vi "HFRR ADV v04.vi"() -> ()   [LabVIEW 2025] (continued)
              n1887 = local write "Com Port 1"(w2844) -> ()
            }
            frame 5 {
              n1888 = local write "visa due"(w2845) -> ()
              n1889 = local write "Com Port 2"(w2845) -> ()
            }
            frame 6 {
              n1890 = String To Path(string=w2846) -> (path=w2847:path)
              n1891 = local write "File Path"(w2847) -> ()
              "String" <- w2846
            }
            frame 7 {
              n1892 = local write "DISPLACEMENT :"(w2848) -> ()
            }
            frame 8 {
              n1893 = local write "STROKE GAIN :"(w2849) -> ()
            }
            frame 9 {
              n1894 = local read "Stroke PID Gains"() -> (w2852:T8)
              n1895 = Bundle By Name(cluster=w2852, "Proportional Gain (Kc)"=w2850) -> (w2851:T8)
              n1896 = local write "Stroke PID Gains"(w2851) -> ()
            }
            frame 10 {
              n1897 = local write "Language Selection"(w2853) -> ()
            }
            frame 11 {
              n1898 = local write "CH-POWER +"(w2854) -> ()
            }
            frame 12 {
              n1899 = local write "CH-POWER -"(w2855) -> ()
            }
            frame 13 {
              n1900 = local write "CH-HEATER"(w2856) -> ()
            }
            frame 14 {
              n1901 = local write "CH-HUMIDITY WET"(w2857) -> ()
            }
            frame 15 {
              n1902 = local write "CH-HUMIDITY DRY"(w2858) -> ()
            }
            frame 16 {
              n1903 = local read "Stroke PID Gains"() -> (w2861:T8)
              n1904 = Bundle By Name(cluster=w2861, "Integral Time (Ti, min)"=w2859) -> (w2860:T8)
              n1905 = local write "Stroke PID Gains"(w2860) -> ()
            }
            frame 17 {
              n1906 = local write "AIR TEMP INTERCEPT:"(w2862) -> ()
            }
            frame 18 {
              n1907 = local write "TEMP INTERCEPT:"(w2863) -> ()
            }
            frame 19 {
              n1908 = local write "S.NO"(w2864) -> ()
            }
            frame 20 {
              n1909 = local write "Com Port 3"(w2865) -> ()
            }
            frame 21 {
              n1910 = local write "LvdtOff"(w2866) -> ()
            }
            frame 22, Default {
            }
          }
        }
      }
    }
    n1911 = case shown="True" w2808 {
      frame False {
        # "79.77669138"
        # "2.3554"
        n1912 = local read "FRIC. FORCE :"() -> (w2871:dbl)
        n1913 = local read "FF cal val"() -> (w2868:dbl[])
        n1914 = Multiply(x=w2871, y=79.77669138) -> (x*y=w2870:dbl)
        n1915 = Multiply(x=w2868, y=w2870) -> (x*y=→"FF Calibration g":dbl[])
        "Err Count" <- 0 ("y")
      }
      frame True {
        n1916 = stacked-sequence {
          frame #0 {
            n1917 = stacked-sequence {
              frame #0 {
                "Lift" <- TRUE ("Lift")
              }
            }
          }
          frame #1 {
            w2883 = 2500 ("y")
            n1918 = local read "FF1"() -> (w2878:dbl[])
            n1919 = local read "Ch1"() -> (w2874:dbl[])
            "Waveform Chart 2" <- w2874
            n1920 = Array Size(array=w2878) -> (size(s)=w2877:i32)
            n1921 = Insert Into Array(array=w2878, index=w2877, new element=w2874) -> (w2880:dbl[])
            n1922 = call-poly <vilib>:"Mean.vi"("X"=w2874) -> ("mean"=→"Raw Mean":dbl)  [unwired: 1 out]
            n1923 = local read "RUN"() -> (w2875:bool)
            n1924 = Array Size(array=w2880) -> (size(s)=w2884:i32)
            n1925 = case shown="False" w2875 {
              frame False {
                n1926 = local write "Frequency"(0.0 ("Frequency")) -> ()
              }
              frame True {
              }
            }
            n1927 = Subtract(x=w2884, y=w2883) -> (x-y=w2882:i32)
            n1928 = Greater?(x=w2884, y=w2883) -> (0:w2885:bool)
            n1929 = case shown="True" w2885 {
              tunnel: w2882 -> [_ w2889]
              tunnel: [w2887 w2891] -> w2876
              tunnel: w2880 -> [w2887 w2890]
              frame False {
              }
              frame True {
                n1930 = Delete From Array(array=w2890, length=w2889, index=0) -> (array with subset deleted=w2891:dbl[])  [unwired: 1 out]
                "Numeric" <- w2889
              }
            }
            "FF1" <- w2876
            "PID Ref" <- TRUE ("PID Ref")
          }
          frame #2 {
          }
          frame #3 {
            w2899 = 0.0 ("lower limit")
            # "CONVERT TO N"
            # "DATA PROCESSING"
            # "115 mV/N"
            n1931 = local read "Fric Val"() -> (w2961:dbl[])
            n1932 = local read "FRIC. FORCE :"() -> (w2954:dbl)
            n1933 = local read "Air temp"() -> (w2955:dbl[])
            n1934 = local read "temp buf"() -> (w2957:dbl[])
            n1935 = call-poly <vilib>:"Mean.vi"("X"=w2955) -> ("mean"=w2923:dbl)  [unwired: 1 out]
            "Raw air temp" <- w2923
            n1936 = Multiply(x=w2961, y=1.0) -> (x*y=w2962:dbl[])
            n1937 = Multiply(x=w2954, y=79.77669138) -> (x*y=w2952:dbl)
            n1938 = call-poly <vilib>:"Mean.vi"("X"=w2957) -> ("mean"=w2925:dbl)  [unwired: 1 out]
            "Raw specimen temp" <- w2925
            n1939 = case shown="0, Default" "Calibrating" {
              tunnel: w2925 -> [w2981 _]
              tunnel: [w2981 w2982] -> w2924
              tunnel: w2923 -> [_ w2982]
              frame 0, Default {
              }
              frame 1 {
              }
            }
            n1940 = Multiply(x=w2962, y=w2952) -> (x*y=w2959:dbl[])
            n1941 = Add(x=w2923, y="Offset Air Temp") -> (x+y=w2918:dbl)
            n1942 = local read "AIR TEMPERATURE :"() -> (w2939:dbl)
            n1943 = local read "TEMPERATURE :"() -> (w2938:dbl)
            n1944 = call-poly <vilib>:"Mean.vi"("X"=w2959) -> ("mean"=w2960:dbl)  [unwired: 1 out]
            n1945 = Subtract(x=w2959, y=w2960) -> (x-y=w2929:dbl[])
            n1946 = case shown="True" "Boolean 4" {
              tunnel: w2924 -> [_ w2988]
              tunnel: "Standard Temp. ( °c )" -> [_ w2987]
              frame False {
              }
              frame True {
                n1947 = local read "Captured Values"() -> (w2985:dbl[][])
                n1948 = local write "Boolean 4"(FALSE ("Boolean 4")) -> ()
                n1949 = Build Array(w2987, w2988) -> (w2986:dbl[])
                n1950 = Build Array (concatenate)(w2985, w2986) -> (w2983:dbl[][])
                n1951 = local write "Captured Values"(w2983) -> ()
              }
            }
            n1952 = local read "AIR TEMP INTERCEPT:"() -> (w2935:dbl)
            n1953 = Multiply(x=w2918, y=w2939) -> (x*y=w2920:dbl)
            n1954 = Absolute Value(x=w2929) -> (abs(x)=w2964:dbl[])
            n1955 = Multiply(x=w2925, y=w2938) -> (x*y=w2919:dbl)
            n1956 = local read "TEMP INTERCEPT:"() -> (w2930:dbl)
            n1957 = local read "RH Numeric:"() -> (w2893:dbl)
            n1958 = call-poly <vilib>:"RMS.vi"("X"=w2929) -> ("rms value"=w2928:dbl)  [unwired: 1 out]
            n1959 = call-poly <vilib>:"Mean.vi"("X"=w2964) -> ()  [unwired: 2 out]
            n1960 = local read "RUN"() -> (w2951:bool)
            n1961 = local read "HUMIDITY:"() -> (w2894:dbl)
            n1962 = Add(x=w2920, y=w2935) -> (x+y=w2937:dbl)
            n1963 = Add(x=w2919, y=w2930) -> (x+y=w2936:dbl)
            n1964 = local read "FRICVALZ"() -> (w2969:dbl)
            n1965 = Multiply(x=w2893, y=w2894) -> (x*y=→"Humidity ( %RH )" →"Hum" →"Hum 2":dbl)
            n1966 = call <vilib>:"Mean PtByPt.vi"("x"=w2936, "sample length"=10) -> ("mean"=w2895:dbl)  [unwired: 2 in, 1 out]
            "TEMP 2" <- w2895
            "TEMP 3" <- w2895
            n1967 = Select(t=0.01 ("FF fil1"), s=w2951, f=0.1 ("FF fil1")) -> (s? t:f=w2947:dbl)
            n1968 = Or(x="FRICVALZ 3", y="FRICVALZ 2") -> (x .or. y?=w2897:bool)
            n1969 = case shown="True" w2897 {
              tunnel: w2928 -> [_ w2993]
              frame False {
              }
              frame True {
                w2992 = FALSE ("FRICVALZ")
                n1970 = local write "FRICVALZ 3"(w2992) -> ()
                n1971 = local write "FRICVALZ 2"(w2992) -> ()
                "FRICVALZ" <- w2993
              }
            }
            n1972 = Subtract(x=w2928, y=w2969) -> (x-y=w2963:dbl)
            n1973 = local read "AIR TEMP"() -> (w2944:dbl)
            n1974 = Multiply(x=w2937, y=w2947) -> (x*y=w2948:dbl)
            n1975 = case shown="True" "Boolean 5" {
              frame False {
              }
              frame True {
                n1976 = local write "Captured Values"(dbl[][] [] ("Captured Values")) -> ()
                n1977 = local write "Boolean 5"(FALSE) -> ()
                n1978 = local write "Best Fit"(dbl[] [] ("Best Fit")) -> ()
              }
            }
            n1979 = local read "FF 2"() -> (w2971:dbl)
            n1980 = Subtract(x=1.0 ("y"), y=w2947) -> (x-y=w2945:dbl)
            n1981 = Multiply(x=w2945, y=w2944) -> (x*y=w2943:dbl)
            n1982 = Multiply(x=w2963, y=0.1 ("FF fil1")) -> (x*y=w2975:dbl)
            n1983 = local write "TEMP"(w2895) -> ()
            n1984 = Multiply(x=0.9 ("FF fil2"), y=w2971) -> (x*y=w2974:dbl)
            n1985 = Add(x=w2948, y=w2943) -> (x+y=w2941:dbl)
            n1986 = local read "ecr buf"() -> (w2916:dbl[])
            n1987 = Add(x=w2975, y=w2974) -> (x+y=w2898:dbl)
            "FF 2" <- w2898
            "FF 4" <- w2898
            n1988 = local read "NORMAL LOAD"() -> (w2958:dbl)
            n1989 = Not A Number/Path/Refnum?(number/path/refnum=w2941) -> (NaN/Path/Refnum?=w2942:bool)
            n1990 = Select(t=0.0, s=w2942, f=w2941) -> (s? t:f=w2901:dbl)
            "AIR TEMP" <- w2901
            n1991 = call-poly <vilib>:"Mean.vi"("X"=w2916) -> ("mean"=w2913:dbl)  [unwired: 1 out]
            n1992 = Multiply(x=w2913, y="ECR_Gain") -> (x*y=w2912:dbl)
            n1993 = local read "TEMP"() -> (w2968:dbl)
            n1994 = local read "ecr"() -> (w2907:dbl)
            n1995 = Divide(x=w2898, y=w2958) -> (x/y=w2931:dbl)
            n1996 = Multiply(x=w2912, y=0.2) -> (x*y=w2905:dbl)
            n1997 = Multiply(x=0.8, y=w2907) -> (x*y=w2906:dbl)
            n1998 = call "Elapsed Time11"("Time Target (s)"=1.0) -> ("Time has Elapsed"=w2903:bool)  [unwired: 11 in, 7 out]
            n1999 = Not A Number/Path/Refnum?(number/path/refnum=w2968) -> (NaN/Path/Refnum?=w2967:bool)
            n2000 = Not A Number/Path/Refnum?(number/path/refnum=w2898) -> (NaN/Path/Refnum?=w2966:bool)
            n2001 = Not A Number/Path/Refnum?(number/path/refnum=w2931) -> (NaN/Path/Refnum?=w2933:bool)
            n2002 = Add(x=w2905, y=w2906) -> (x+y=w2904:dbl)
            n2003 = Select(t=0.0, s=w2933, f=w2931) -> (s? t:f=→"COF 2":dbl)
            n2004 = case shown="True" w2903 {
              tunnel: w2901 -> [_ w2977]
              frame False {
              }
              frame True {
                "AirT" <- w2977
              }
            }
            n2005 = Compound Arithmetic op=OR(w2967, w2966) -> (w2965:bool)
            n2006 = Not A Number/Path/Refnum?(number/path/refnum=w2904) -> (NaN/Path/Refnum?=w2914:bool)
            n2007 = case shown="True" w2965 {
              frame False {
              }
              frame True {
                n2008 = local write "TEMP"(0.0 ("TEMP")) -> ()
                n2009 = local write "reinit"(TRUE ("reinit")) -> ()
                n2010 = local write "FF 2"(0.0 ("FF 2")) -> ()
              }
            }
            n2011 = Select(t=0.0, s=w2914, f=w2904) -> (s? t:f=w2911:dbl)
            n2012 = In Range and Coerce(upper limit=100.0, x=w2911, lower limit=w2899) -> ()  [unwired: 2 out]
            "ecr" <- w2899
          }
          frame #4 {
            n2013 = case shown="True" "Boolean 6" {
              frame False {
              }
              frame True {
                n2014 = local read "Captured Values"() -> (w3004:dbl[][])
                n2015 = Index Array(array=w3004, index (col) #1=0 ("disabled index (col)"), index (col) #2=1 ("index (col)")) -> (element #1=w3002:dbl[], element #2=w3000:dbl[])  [unwired: 2 in]
                n2016 = local write "Boolean 6"(FALSE ("Boolean 6")) -> ()
                n2017 = call <vilib>:"Linear Fit.vi"("Y"=w3002, "X"=w3000) -> ("Best Linear Fit"=→"Best Fit":dbl[], "slope"=w2996:dbl, "intercept"=w2995:dbl)  [unwired: 9 in, 2 out]
                "Slope" <- w2996
                "Intercept" <- w2995
                n2018 = local read "Calibrating"() -> (w2997:u16)
                n2019 = case shown="1" w2997 {
                  tunnel: w2996 -> [w3006 w3008]
                  tunnel: w2995 -> [w3005 w3007]
                  frame 0, Default {
                    n2020 = local write "TEMPERATURE :"(w3006) -> ()
                    n2021 = local write "TEMP INTERCEPT:"(w3005) -> ()
                  }
                  frame 1 {
                    n2022 = local write "AIR TEMPERATURE :"(w3008) -> ()
                    n2023 = local write "AIR TEMP INTERCEPT:"(w3007) -> ()
                  }
                }
              }
            }
            n2024 = flat-sequence {
              frame #0 {
                n2025 = Wait (ms)(milliseconds to wait=u32 100) -> ()  [unwired: 1 out]
              }
              frame #1 {
                n2026 = local write "Lift"(FALSE ("Lift")) -> ()
              }
            }
          }
        }
      }
    }
    n2027 = local read "EXIT"() -> (w2815:bool)
    "Rate" <- 2500.0 ("No of Samples")
    "Humid Last buf" <- dbl[] [0.0, 0.0, 0.0, 0.0] ("Humid Last buf")
  }
  n2028 = VISA Close(VISA resource name=w13, error in (no error)=w12) -> (error out=w14:errorcluster)
  n2029 = call <vilib>:"Clear Errors.vi"("error in (no error)"=w14) -> ()  [unwired: 5 in, 2 out]
  n2030 = VISA Close(VISA resource name=w36, error in (no error)=w35) -> (error out=w33:errorcluster)
  n2031 = call <vilib>:"Clear Errors.vi"("error in (no error)"=w33) -> ()  [unwired: 5 in, 2 out]
  n2032 = Or(x=w23, y=w22) -> (x .or. y?=w24:bool)
  n2033 = while {
    tunnel: [w3070] -> w29
    shift-right: [w3050] -> _
    shift-left: "" -> [w3038]
    tunnel: [w3026] -> _
    i -> [w3026]
    stop <- w3070 stop-if-true
    w3052 = ";" ("string")
    n2034 = local read "start en"() -> (w3072:bool)
    n2035 = And(x="st enable", y=w3072) -> (x .and. y?=w3073:bool)
    n2036 = local read "ACQUIRE 3"() -> (w3015:bool)
    n2037 = local read "Elapsed time"() -> (w3034:dbl)
    n2038 = case shown="True" w3073 {
      tunnel: "st enable" -> [w3137 w3138]
      tunnel: [w3137 w3138] -> w3016
      frame False {
      }
      frame True {
        n2039 = local write "start en"(FALSE ("start en")) -> ()
      }
    }
    n2040 = Wait (ms)(milliseconds to wait=u32 80) -> ()  [unwired: 1 out]
    n2041 = local read "Stroke"() -> (w3025:dbl)
    n2042 = Greater?(x=w3034, y=0.1) -> (0:w3032:bool)
    n2043 = Or(x=w3016, y=w3015) -> (x .or. y?=w3017:bool)
    n2044 = case shown="True" "ACQUIRE 2" {
      frame False {
      }
      frame True {
        n2045 = call "Elapsed Time13"() -> ("Time has Elapsed"=w3080:bool)  [unwired: 12 in, 7 out]
        n2046 = case shown="True" w3080 {
          frame False {
          }
          frame True {
            n2047 = local write "ACQUIRE 2"(FALSE ("ACQUIRE 2")) -> ()
            n2048 = local write "ACQUIRE 3"(FALSE ("ACQUIRE 2")) -> ()
          }
        }
        n2049 = local write "ACQUIRE 3"(TRUE ("ACQUIRE 2")) -> ()
      }
    }
    n2050 = case shown="True" w3017 {
      tunnel: w3025 -> [_ w3160]
      tunnel: [w3140 _] -> w3069
      tunnel: w3032 -> [_ _]
      tunnel: w3015 -> [_ w3147]
      frame False {
        w3140 = TRUE ("PID Rst")
        n2051 = local read "stop cmd"() -> (w3141:bool)
        n2052 = case shown="True" w3141 {
          frame False {
          }
          frame True {
            n2053 = local write "stop cmd"(FALSE ("stop cmd")) -> ()
          }
        }
        n2054 = local write "PID Rst"(TRUE ("PID Rst")) -> ()
        "start en" <- w3140
      }
      frame True {
        w3167 = cluster{"output high":dbl, "output low":dbl} {"output high"=600.0, "output low"=-600.0} ("output range")
        n2055 = local read "STROKE GAIN :"() -> (w3152:dbl)
        n2056 = call "Elapsed Time6"("Reset"="PID Rst", "Auto Reset"=FALSE) -> ("Time has Elapsed"=w3161:bool)  [unwired: 10 in, 7 out]
        n2057 = Multiply(x="Set Strk", y=w3152) -> (x*y=w3145:dbl)
        n2058 = case shown="False" w3161 {
          tunnel: [w3172 w3173] -> w3164
          tunnel: "Set Strk" -> [w3172 _]
          tunnel: w3160 -> [_ w3173]
          frame False {
          }
          frame True {
          }
        }
        n2059 = Multiply(x=w3145, y=1.0) -> (x*y=w3144:dbl)
        n2060 = Select(t=T8 {"Proportional Gain (Kc)"=0.0, "Integral Time (Ti, min)"=0.02, "Derivative Time (Td, min)"=0.0} ("Stroke PID Gains"), s=w3147, f="Stroke PID Gains") -> (s? t:f=w3148:T8)
        n2061 = Not(x=w3161) -> (.not. x?=w3159:bool)
        n2062 = call-poly <vilib>:"PID.vi"("reinitialize? (F)"=w3159, "output range"=w3167, "PID gains"=w3148, "process variable"=w3164, "setpoint"="Set Strk") -> ("output"=w3158:dbl)  [unwired: 5 in, 1 out]
        "Slide 5" <- w3158
        n2063 = Select(t=w3158, s=w3161, f=0.0) -> (s? t:f=w3162:dbl)
        n2064 = flat-sequence {
          tunnel: w3162 -> [_]
          frame #0 {
            n2065 = local write "PID Rst"(FALSE ("PID Rst")) -> ()
          }
        }
        n2066 = Add(x=w3144, y=w3162) -> (x+y=w3157:dbl)
        n2067 = Unbundle(w3167) -> ("output high"=w3166:dbl, "output low"=w3165:dbl)
        n2068 = To Word Integer(number=w3157) -> (16bit integer=w3154:i16)
        n2069 = property on="Slide 5" class="Slide (strict)"("Scale.Range:Minimum"=w3165, "Scale.Range:Maximum"=w3166) -> ()  [unwired: 2 in, 2 out]
        n2070 = In Range and Coerce(upper limit=4095.0 ("f"), x=w3154, lower limit=100.0 ("f")) -> (coerced(x)=w3151:dbl)  [unwired: 1 out]
        "PID Out" <- w3151
        n2071 = Number To Decimal String(number=w3151) -> (decimal integer string=→"st gain":string)  [unwired: 1 in]
        "stop cmd" <- TRUE ("Auto Reset")
      }
    }
    n2072 = flat-sequence {
      frame #0 {
        n2073 = local read "CH-POWER +"() -> (w3084:u16)
        n2074 = local read "CH-POWER -"() -> (w3085:u16)
        n2075 = case shown="1" w3085 {
          tunnel: "PWR" -> [w3086 w3087 w3088 w3089 w3090 w3091 w3092 w3093]
          frame 0, Default {
            n2076 = local write "Do 0"(w3086) -> ()
          }
          frame 1 {
            n2077 = local write "Do 1"(w3087) -> ()
          }
          frame 2 {
            n2078 = local write "Do 2"(w3088) -> ()
          }
          frame 3 {
            n2079 = local write "Do 3"(w3089) -> ()
          }
          frame 4 {
            n2080 = local write "Do 4"(w3090) -> ()
          }
          frame 5 {
            n2081 = local write "Do 5"(w3091) -> ()
          }
          frame 6 {
            n2082 = local write "Do 6"(w3092) -> ()
          }
          frame 7 {
            n2083 = local write "Do 7"(w3093) -> ()
          }
        }
        n2084 = case shown="1" w3084 {
          tunnel: "PWR" -> [w3094 w3095 w3096 w3097 w3098 w3099 w3100 w3101]
          frame 0, Default {
            n2085 = local write "Do 0"(w3094) -> ()
          }
          frame 1 {
            n2086 = local write "Do 1"(w3095) -> ()
          }
          frame 2 {
            n2087 = local write "Do 2"(w3096) -> ()
          }
          frame 3 {
            n2088 = local write "Do 3"(w3097) -> ()
          }
          frame 4 {
            n2089 = local write "Do 4"(w3098) -> ()
          }
          frame 5 {
            n2090 = local write "Do 5"(w3099) -> ()
          }
          frame 6 {
            n2091 = local write "Do 6"(w3100) -> ()
          }
          frame 7 {
            n2092 = local write "Do 7"(w3101) -> ()
          }
        }
      }
    }
    n2093 = local read "RUN"() -> (w3023:bool)
    n2094 = Or(x=w3023, y="ACQUIRE 3") -> (x .or. y?=w3022:bool)
    n2095 = local read "Set Hz"() -> (w3040:dbl)
    n2096 = Select(t=w3040, s=w3022, f=0.0) -> (s? t:f=w3039:dbl)
    n2097 = local read "st gain"() -> (w3043:string)
    n2098 = local read "DO"() -> (w3044:string)
    n2099 = case shown="True" "Boolean 10" {
      frame False {
      }
      frame True {
        n2100 = local write "Tab Control 8"(enum32{"setup", "calibrate"}."calibrate" ("Tab Control 8")) -> ()
        n2101 = local write "Boolean 10"(FALSE ("Boolean 10")) -> ()
      }
    }
    n2102 = Number To Decimal String(number=w3039) -> (decimal integer string=w3042:string)  [unwired: 1 in]
    n2103 = case shown="True" "Boolean 11" {
      frame False {
      }
      frame True {
        n2104 = local write "Tab Control 8"(enum32{"setup", "calibrate"}."setup" ("Tab Control 8")) -> ()
        n2105 = local write "Boolean 11"(FALSE ("Boolean 11")) -> ()
      }
    }
    n2106 = String Length(string=w3043) -> (length=w3058:i32)
    n2107 = String Length(string=w3044) -> (length=w3046:i32)
    n2108 = String Length(string=w3042) -> (length=w3059:i32)
    n2109 = Subtract(x=4.0, y=w3058) -> (x-y=w3055:dbl)
    n2110 = Subtract(x=3.0, y=w3046) -> (x-y=w3049:dbl)
    n2111 = flat-sequence {
      tunnel: w3069 -> [_]
      frame #0 {
        n2112 = Build Array("Do 0", "Do 1", "Do 2", "Do 3", "Do 4", "Do 5", "Do 6", "Do 7") -> (w3128:bool[])
        n2113 = Boolean Array To Number(Boolean array=w3128) -> (number=w3126:u32)
        n2114 = Add(x=w3126, y=u32 0) -> (x+y=w3124:u32)
        n2115 = Number To Decimal String(number=w3124) -> (decimal integer string=→"DO":string)  [unwired: 1 in]
      }
    }
    n2116 = Subtract(x=3.0, y=w3059) -> (x-y=w3060:dbl)
    n2117 = Replace Substring(3:w3055, 4:w3043, 5:"0000" ("string")) -> (1:w3053:string)  [unwired: 1 in, 1 out]
    n2118 = Replace Substring(3:w3049, 4:w3044, 5:"000" ("string")) -> (1:w3045:string)  [unwired: 1 in, 1 out]
    n2119 = Replace Substring(3:w3060, 4:w3042, 5:"000" ("string")) -> (1:w3054:string)  [unwired: 1 in, 1 out]
    n2120 = Concatenate Strings("*" ("string"), w3054, w3052, w3053, w3052, w3045, "$" ("string")) -> (w3050:string)
    "Stroke_send_Val" <- w3050
    n2121 = local read "RUN"() -> (w3020:bool)
    n2122 = local read "ACQUIRE 3"() -> (w3019:bool)
    n2123 = local read "send"() -> (w3036:bool)
    n2124 = Not Equal?(x=w3038, y=w3050) -> (x != y?=w3051:bool)
    n2125 = Or(x=w3020, y=w3019) -> (x .or. y?=w3018:bool)
    n2126 = And(x=w3036, y=w3018) -> (x .and. y?=w3035:bool)
    n2127 = Or(x=w3051, y=w3035) -> (x .or. y?=w3029:bool)
    n2128 = case shown="False" w3018 {
      frame False {
        "send" <- TRUE ("send")
      }
      frame True {
      }
    }
    n2129 = call "Elapsed Time4"("Time Target (s)"=0.5) -> ("Time has Elapsed"=w3027:bool)  [unwired: 11 in, 7 out]
    n2130 = local read "Din"() -> (w3068:u8[])
    n2131 = Or(x=w3027, y=w3029) -> (x .or. y?=w3028:bool)
    n2132 = Index Array(array=w3068, index=0) -> (element=w3066:u8)
    n2133 = case shown="True" w3028 {
      tunnel: w3050 -> [_ w3105]
      frame False {
      }
      frame True {
        n2134 = local read "Due Com"() -> (w3106:string[])
        n2135 = Build Array (concatenate)(w3106, w3105) -> (→"Due Com":string[])
        n2136 = local write "send"(FALSE ("send")) -> ()
      }
    }
    n2137 = Number To Boolean Array(number=w3066) -> (Boolean array=w3065:bool[])
    n2138 = Array Size(array=w3065) -> (size(s)=w3064:i32)
    n2139 = Greater Than 0?(x=w3064) -> (x > 0?=w3063:bool)
    n2140 = case shown="True" w3063 {
      tunnel: w3065 -> [_ w3120]
      frame False {
      }
      frame True {
        n2141 = Index Array(array=w3120, index #1=0 ("index"), index #2=1 ("index"), index #3=2 ("index"), index #4=3 ("index"), index #5=4 ("index"), index #6=5 ("index"), index #7=6 ("index"), index #8=7 ("index")) -> (element #1=→"DI 0":bool, element #2=→"DI 1":bool, element #3=→"DI 2":bool, element #4=→"DI 3":bool, element #5=→"DI 4":bool, element #6=→"DI 5":bool, element #7=→"DI 6":bool, element #8=→"DI 7":bool)
      }
    }
    n2142 = local read "EXIT"() -> (w3070:bool)
  }
  n2143 = Or(x=w17, y=w24) -> (x .or. y?=w31:bool)
  n2144 = control-ref of="new picture"() -> ()  [unwired: 1 out]
  n2145 = Or(x=w38, y=w31) -> (x .or. y?=w28:bool)
  n2146 = Or(x=w28, y=w29) -> (x .or. y?=w19:bool)
  n2147 = while {
    tunnel: w15 -> [_]
    tunnel: [w3176] -> w42
    tunnel: [w3175] -> _
    i -> [w3175]
    stop <- w3176 stop-if-true
    n2148 = local read "PID-out"() -> (w3177:dbl)
    "Horizontal Slider Control" <- w3177
    n2149 = Greater Or Equal?(x=w3177, y=2.0) -> (x >= y?=w3178:bool)
    n2150 = flat-sequence {
      tunnel: w3178 -> [w3186]
      tunnel: w3177 -> [w3189]
      tunnel: [w3187] -> w3184
      tunnel: [w3185] -> w3183
      tunnel: [w3205] -> w3182
      tunnel: w3184 -> [w3205]
      tunnel: w3183 -> [w3202]
      tunnel: [w3202] -> w3181
      tunnel: w3182 -> [w3207]
      tunnel: [w3206] -> w3180
      tunnel: w3181 -> [w3206]
      tunnel: w3180 -> [w3221]
      frame #0 {
        n2151 = case shown="True" w3186 {
          selector: w3186 -> [w3191 _]
          frame False {
            n2152 = local write "HEATER"(w3191) -> ()
          }
          frame True {
            w3193 = TRUE ("data")
            n2153 = local read "CH-HEATER"() -> (w3192:u16)
            n2154 = case shown="2" w3192 {
              tunnel: w3193 -> [w3194 w3195 w3196 w3197 w3198 w3199 w3200 w3201]
              frame 0, Default {
                n2155 = local write "Do 0"(w3194) -> ()
              }
              frame 1 {
                n2156 = local write "Do 1"(w3195) -> ()
              }
              frame 2 {
                n2157 = local write "Do 2"(w3196) -> ()
              }
              frame 3 {
                n2158 = local write "Do 3"(w3197) -> ()
              }
              frame 4 {
                n2159 = local write "Do 4"(w3198) -> ()
              }
              frame 5 {
                n2160 = local write "Do 5"(w3199) -> ()
              }
              frame 6 {
                n2161 = local write "Do 6"(w3200) -> ()
              }
              frame 7 {
                n2162 = local write "Do 7"(w3201) -> ()
              }
            }
            "HEATER" <- w3193
          }
        }
        n2163 = Select(t=w3189, s=w3186, f=0.0) -> (s? t:f=w3185:dbl)
        n2164 = Greater Or Equal?(x=w3189, y=97.0) -> (x >= y?=w3187:bool)
      }
      frame #1 {
        n2165 = Multiply(x=w3202, y=5.0) -> (x*y=w3204:dbl)
        n2166 = Wait (ms)(milliseconds to wait=w3204) -> ()  [unwired: 1 out]
      }
      frame #2 {
        n2167 = case shown="True" w3207 {
          frame False {
            w3208 = FALSE ("data")
            n2168 = local write "HEATER"(w3208) -> ()
            n2169 = local read "CH-HEATER"() -> (w3209:u16)
            n2170 = case shown="4" w3209 {
              tunnel: w3208 -> [w3210 w3211 w3212 w3213 w3214 w3215 w3216 w3217]
              frame 0, Default {
                n2171 = local write "Do 0"(w3210) -> ()
              }
              frame 1 {
                n2172 = local write "Do 1"(w3211) -> ()
              }
              frame 2 {
                n2173 = local write "Do 2"(w3212) -> ()
              }
              frame 3 {
                n2174 = local write "Do 3"(w3213) -> ()
              }
              frame 4 {
                n2175 = local write "Do 4"(w3214) -> ()
              }
              frame 5 {
                n2176 = local write "Do 5"(w3215) -> ()
              }
              frame 6 {
                n2177 = local write "Do 6"(w3216) -> ()
              }
              frame 7 {
                n2178 = local write "Do 7"(w3217) -> ()
              }
            }
          }
          frame True {
          }
        }
      }
      frame #3 {
        n2179 = Subtract(x=100, y=w3221) -> (x-y=w3220:dbl)
        n2180 = Multiply(x=w3220, y=5.0) -> (x*y=w3218:dbl)
        n2181 = Wait (ms)(milliseconds to wait=w3218) -> ()  [unwired: 1 out]
      }
    }
    n2182 = local read "EXIT"() -> (w3176:bool)
  }
  n2183 = disable-structure shown="Disabled" {
    disable-tunnel: [w3229 _] -> w20
    frame Disabled {
      n2184 = while {
        shift-right: [w3271] -> w3227
        shift-left: errorcluster {"status"=TRUE, "code"=0, "source"="Init"} ("error out") -> [w3235]
        shift-right: [w3270] -> w3226
        shift-left: _ -> [w3236]
        shift-right: [w3269] -> _
        shift-left: "" -> [w3268]
        tunnel: [w3267] -> w3229
        shift-right: ["Set Rh"] -> _
        shift-left: 0.0 ("Set Rh") -> [w3261]
        tunnel: [w3238] -> _
        i -> [w3238]
        stop <- w3267 stop-if-true
        n2185 = flat-sequence {
          tunnel: w3235 -> [w3274]
          tunnel: [w3274] -> w3234
          frame #0 {
            n2186 = Wait (ms)(milliseconds to wait=u32 200) -> ()  [unwired: 1 out]
          }
        }
        n2187 = local read "Com Port 3"() -> (w3237:refnum<visa-resource-name>)
        n2188 = local read "Humidity Str Rec"() -> (w3239:string)
        n2189 = Not Equal?(x="Set Rh", y=w3261) -> (x != y?=w3266:bool)
        n2190 = Number To Decimal String(number="Set Rh") -> (decimal integer string=w3264:string)  [unwired: 1 in]
        n2191 = Not Equal?(x=w3237, y=w3236) -> (x != y?=w3232:bool)
        n2192 = Concatenate Strings("#setPoint00" ("string"), w3264) -> (w3265:string)
        n2193 = case shown="False" w3266 {
          tunnel: w3265 -> [_ w3286]
          frame False {
            n2194 = local read "Humidity"() -> (w3283:bool)
            n2195 = case shown="True" w3283 {
              frame False {
                n2196 = local write "Humidity Str Send"("stop" ("Humidity Str Send")) -> ()
              }
              frame True {
                n2197 = local write "Humidity Str Send"("start" ("Humidity Str Send")) -> ()
              }
            }
          }
          frame True {
            n2198 = local write "Humidity Str Send"(w3286) -> ()
          }
        }
        n2199 = Or(x=w3232, y="Re-Initialise") -> (x .or. y?=w3231:bool)
        n2200 = String Subset(string=w3239, offset (0)=7) -> (substring=w3254:string)  [unwired: 1 in]
        n2201 = Match Pattern(string=w3239, regular expression="?") -> (offset past match=w3257:i32)  [unwired: 1 in, 3 out]
        n2202 = Match Pattern(string=w3239, regular expression="v") -> (offset past match=w3260:i32)  [unwired: 1 in, 3 out]
        n2203 = case shown="True" w3231 {
          tunnel: w3234 -> [w3272 _]
          tunnel: [w3272 errorcluster {"status"=TRUE, "code"=0, "source"="Init"} ("error out")] -> w3233
          frame False {
          }
          frame True {
          }
        }
        n2204 = Equal?(x=w3257, y=-1) -> (x = y?=w3241:bool)
        n2205 = Match Pattern(string=w3254, regular expression="g") -> (after substring=w3255:string, offset past match=w3246:i32)  [unwired: 1 in, 2 out]
        n2206 = Match Pattern(string=w3254, regular expression="y") -> (after substring=w3253:string, offset past match=w3247:i32)  [unwired: 1 in, 2 out]
        n2207 = Greater?(x=w3247, y=w3246) -> (0:w3252:bool)
        n2208 = Greater Or Equal To 0?(x=w3247) -> (x >= 0?=w3244:bool)
        n2209 = Greater Or Equal To 0?(x=w3246) -> (x >= 0?=w3245:bool)
        n2210 = Or(x=w3244, y=w3245) -> (x .or. y?=w3243:bool)
        n2211 = Greater Or Equal To 0?(x=w3260) -> (x >= 0?=w3242:bool)
        n2212 = Select(t=w3253, s=w3252, f=w3255) -> (s? t:f=w3248:string)
        n2213 = case shown="Error" w3233 {
          selector: w3233 -> [w3299 w3345]
          tunnel: [w3297 w3338] -> w3271
          tunnel: w3236 -> [w3300 w3344]
          tunnel: [w3298 w3347] -> w3270
          tunnel: w3268 -> [w3287 w3346]
          tunnel: [w3294 w3346] -> w3269
          frame No Error {
            n2214 = call "Elapsed Time7"() -> ("Time has Elapsed"=w3293:bool)  [unwired: 12 in, 7 out]
            n2215 = Not Equal?(x="Humidity Str Send", y=w3287) -> (x != y?=w3289:bool)
            n2216 = Or(x=w3289, y=w3293) -> (x .or. y?=w3292:bool)
            n2217 = Select(t="Humidity Str Send", s=w3289, f="vals" ("regular expression")) -> (s? t:f=w3288:string)
            n2218 = Or(x=w3292, y="Send") -> (x .or. y?=w3296:bool)
            n2219 = case shown="True" w3296 {
              tunnel: [w3303 w3308] -> w3297
              tunnel: w3300 -> [w3302 w3316]
              tunnel: w3299 -> [w3303 w3315]
              tunnel: [w3302 w3309] -> w3298
              tunnel: w3288 -> [_ w3314]
              tunnel: [w3301 w3305] -> w3294
              tunnel: "Humidity Str Send" -> [_ w3306]
              tunnel: w3289 -> [_ w3307]
              tunnel: w3287 -> [w3301 w3304]
              frame False {
              }
              frame True {
                n2220 = Select(t=w3306, s=w3307, f=w3304) -> (s? t:f=w3305:string)
                n2221 = flat-sequence {
                  tunnel: w3316 -> [w3324]
                  tunnel: w3315 -> [w3323]
                  tunnel: w3314 -> [w3320]
                  tunnel: [w3322] -> w3313
                  tunnel: [w3321] -> w3312
                  tunnel: w3313 -> [w3327]
                  tunnel: w3312 -> [w3326]
                  tunnel: [w3327] -> w3311
                  tunnel: [w3326] -> w3310
                  tunnel: w3311 -> [w3334]
                  tunnel: w3310 -> [w3333]
                  tunnel: [w3332] -> w3309
                  tunnel: [w3331] -> w3308
                  frame #0 {
                    n2222 = local write "Ser Led"(TRUE ("Boolean 4")) -> ()
                    n2223 = Concatenate Strings(w3320, "\r") -> (w3319:string)
                    n2224 = VISA Write(VISA resource name=w3324, write buffer=w3319, error in (no error)=w3323) -> (VISA resource name out=w3322:refnum<visa-resource-name>, error out=w3321:errorcluster)  [unwired: 1 out]
                  }
                  frame #1 {
                    n2225 = Wait (ms)(milliseconds to wait="wait") -> ()  [unwired: 1 out]
                  }
                  frame #2 {
                    w3329 = FALSE ("Send")
                    n2226 = property class="Instr"(reference=w3334, error in=w3333) -> (reference out=w3335:refnum<visa-resource-name>, error out=w3336:errorcluster, "Serial Settings:Number of Bytes at Serial Port"=w3328:u32)
                    "Humidity 2" <- w3328
                    n2227 = local write "Send"(w3329) -> ()
                    n2228 = local write "Ser Led"(w3329) -> ()
                    n2229 = VISA Read(VISA resource name=w3335, byte count=w3328, error in (no error)=w3336) -> (VISA resource name out=w3332:refnum<visa-resource-name>, read buffer=→"Humidity Str Rec":string, error out=w3331:errorcluster)  [unwired: 1 out]
                  }
                }
              }
            }
          }
          frame Error {
            w3352 = u16 0 items=["None"=0, "XON/XOFF"=1, "RTS/CTS"=2, "DTR/DSR"=4] ("flow control")
            w3348 = u16 0 items=["None", "Odd", "Even", "Mark", "Space"] ("parity")
            w3351 = u16 10 items=["1.0"=10, "1.5"=15, "2.0"=20] ("stop bits")
            n2230 = VISA Close(VISA resource name=w3344, error in (no error)=w3345) -> (error out=w3343:errorcluster)
            n2231 = local write "humid"("" ("humid")) -> ()
            n2232 = local write "Humidity Str Rec"("" ("Humidity Str Rec")) -> ()
            n2233 = call <vilib>:"Clear Errors.vi"("error in (no error)"=w3343) -> ("error out"=w3342:errorcluster)  [unwired: 5 in, 1 out]
            n2234 = local read "Com Port 3"() -> (w3341:refnum<visa-resource-name>)
            n2235 = call-poly "VISA Configure Serial Port"("VISA resource name"=w3341, "timeout (10sec)"=u32 1000, "termination char\n(0xA = '\\n' = LF)"=u8 10 ("termination char\n(0xA = '\\n' = LF)"), "Enable Termination\nChar (T)"=FALSE ("Enable Termination Char (T)"), "baud rate (9600)"="Humidity BaudRate", "data bits (8)"=u16 8 ("data bits"), "parity (0:none)"=w3348, "error in (no error)"=w3342, "stop bits (10: 1 bit)"=w3351, "flow control (0:none)"=w3352) -> ("VISA resource name out"=w3347:refnum<visa-resource-name>, "error out"=w3338:errorcluster)  [unwired: 4 in]
          }
        }
        n2236 = Compound Arithmetic op=AND(w3242, w3241, w3243) -> (w3240:bool)
        n2237 = case shown="True" w3240 {
          tunnel: w3239 -> [_ _]
          tunnel: w3248 -> [_ w3279]
          frame False {
          }
          frame True {
            w3277 = " " ("regular expression")
            n2238 = Match Pattern(string=w3279, regular expression=" ") -> (after substring=w3281:string)  [unwired: 1 in, 3 out]
            n2239 = Match Pattern(string=w3281, regular expression=w3277) -> (before substring=→"humid":string, after substring=w3278:string)  [unwired: 1 in, 2 out]
            n2240 = Match Pattern(string=w3278, regular expression=w3277) -> (before substring=→"temp_@Rh sensor":string)  [unwired: 1 in, 3 out]
          }
        }
        n2241 = local read "EXIT"() -> (w3267:bool)
      }
      n2242 = VISA Close(VISA resource name=w3226, error in (no error)=w3227) -> (error out=w3223:errorcluster)
      n2243 = call <vilib>:"Clear Errors.vi"("error in (no error)"=w3223) -> ()  [unwired: 5 in, 2 out]
    }
    frame Enabled {
    }
  }
  n2244 = Or(x=w19, y=w20) -> (x .or. y?=w18:bool)
  n2245 = Or(x=w42, y=w18) -> (x .or. y?=w41:bool)
  n2246 = while {
    tunnel: [w3360] -> _
    tunnel: w15 -> [_]
    i -> [w3360]
    stop <- w3359 stop-if-true
    # "Langauage selection"
    n2247 = property on="FF Calibration g" class="WFGraph (strict)"("Plot Area:Colors:FG Color"=u32 0) -> ()  [unwired: 2 in, 2 out]
    n2248 = Equal?(x="Lan flag", y=22.0) -> ()  [unwired: 1 out]
    n2249 = disable-structure shown="Disabled" {
      frame Disabled {
        n2250 = stacked-sequence {
          frame #0 {
            n2251 = case shown="\"Russian\"" "Language Selection" {
              tunnel: [0 1] -> w3362
              frame "English", Default {
              }
              frame "Russian" {
              }
            }
            n2252 = for {
              N: 130 -> [_]
              tunnel: "Table" -> [w3371]
              tunnel: w3362 -> [w3370]
              i -> [w3369]
              n2253 = Index Array(array=w3371, index (row)=w3369, index (col)=w3370) -> (element=w3368:string)
              n2254 = case shown="8" w3369 {
                tunnel: w3368 -> [w3372 w3373 w3374 w3375 w3376 w3377 w3378 w3379 w3380 w3381 w3382 w3383 w3384 w3385 w3386 w3387 w3388 w3389 w3390 w3391 w3392 w3393 w3394 w3395 w3396 w3397 w3398 w3399 w3400 _ _ w3401 w3402 w3403 w3404 w3405 w3406 w3415 w3422 w3429 w3436 w3440 w3443 w3446 w3448 w3450 w3451 w3452 w3453 w3454 w3455 w3456 w3457 w3458 w3459 w3460 w3461 w3462 w3463 w3464 w3465 w3466 w3467 w3468 w3469 w3470 w3471 w3472 w3473 w3474 w3475 w3476 w3477 w3478 w3479 w3480 w3481 w3482 w3483 w3484 w3485 w3486 w3487 w3488 w3489 w3490 w3491 w3492 w3493 w3494 w3495 w3496 w3497 w3498 w3499 w3500 w3501 w3502 w3503 w3504 w3505 w3506 w3507 w3508 w3509 _ w3510 w3511 w3512 w3513 w3514 w3515 w3516 w3517 w3518 w3519 w3520 w3521 w3522 _ w3523 w3524 w3525 w3526 w3527 w3528 _]
                frame 0 {
                  n2255 = local write "S"(w3372) -> ()
                }
                frame 1 {
                  n2256 = local write "S 2"(w3373) -> ()
                }
                frame 2 {
                  n2257 = property on="EXIT" class="Bool (strict)"("Boolean Text.Text"=w3374) -> ()  [unwired: 2 in, 2 out]
                }
                frame 3 {
                  n2258 = local write "S 4"(w3375) -> ()
                }
                frame 4 {
                  n2259 = property on="FILE" class="Str"("Caption.Text"=w3376) -> ()  [unwired: 2 in, 2 out]
                }
                frame 5 {
                  n2260 = property on="Fuel Discription :" class="Str"("Caption.Text"=w3377) -> ()  [unwired: 2 in, 2 out]
                }
                frame 6 {
                  n2261 = property on="Remarks :" class="Str"("Caption.Text"=w3378) -> ()  [unwired: 2 in, 2 out]
                }
                frame 7 {
                  n2262 = property on="Save & Continue" class="Bool (strict)"("Boolean Text.Text"=w3379) -> ()  [unwired: 2 in, 2 out]
                }
                frame 8 {
                  n2263 = property on="STOP 3" class="Bool (strict)"("Boolean Text.Text"=w3380) -> ()  [unwired: 2 in, 2 out]
                }
                frame 9 {
                  n2264 = property on="Set Hz" class="DigNum (strict)"("Caption.Text"=w3381) -> ()  [unwired: 2 in, 2 out]
                }
                frame 10 {
                  "String 3" <- w3382
                }
                frame 11 {
                  n2265 = property on="NORMAL LOAD" class="DigNum (strict)"("Caption.Text"=w3383) -> ()  [unwired: 2 in, 2 out]
                }
                frame 12 {
                  "String 5" <- w3384
                }
                frame 13 {
                  n2266 = property on="Set Temp" class="DigNum (strict)"("Caption.Text"=w3385) -> ()  [unwired: 2 in, 2 out]
                }
                frame 14 {
                  n2267 = local write "S 15"(w3386) -> ()
                }
                frame 15 {
                  n2268 = property on="Set Rh" class="DigNum (strict)"("Caption.Text"=w3387) -> ()  [unwired: 2 in, 2 out]
                }
                frame 16 {
                  "String 13" <- w3388
                  "String 26" <- w3388
                }
                frame 17 {
                  n2269 = local write "S 18"(w3389) -> ()
                }
                frame 18 {
                  "String 17" <- w3390
                }
                frame 19 {
                  n2270 = property on="test time" class="DigNum (strict)"("Caption.Text"=w3391) -> ()  [unwired: 2 in, 2 out]
                }
                frame 20 {
                  "String 18" <- w3392
                  "String 22" <- w3392
                }
                frame 21 {
                  n2271 = property on="Elapsed time" class="DigNum (strict)"("Caption.Text"=w3393) -> ()  [unwired: 2 in, 2 out]
                }
                frame 22 {
                  n2272 = property on="Samplingtime 2" class="DigNum (strict)"("Caption.Text"=w3394) -> ()  [unwired: 2 in, 2 out]
                }
                frame 23 {
                  "String 21" <- w3395
                }
                frame 24 {
                  n2273 = property on="Countdown" class="DigNum (strict)"("Caption.Text"=w3396) -> ()  [unwired: 2 in, 2 out]
                }
                frame 25 {
                  n2274 = property on="Countdown 2" class="DigNum (strict)"("Caption.Text"=w3397) -> ()  [unwired: 2 in, 2 out]
                }
                frame 26 {
                  n2275 = property on="Engage" class="Bool (strict)"("Boolean Text.Text"=w3398) -> ()  [unwired: 2 in, 2 out]
                }
                frame 27 {
                  n2276 = property on="Boolean  4" class="Bool (strict)"("Boolean Text.Text"=w3399) -> ()  [unwired: 2 in, 2 out]
                }
                frame 28 {
                  n2277 = property on="Test \nStatus" class="Bool (strict)"("Boolean Text.Text"=w3400) -> ()  [unwired: 2 in, 2 out]
                }
                frame 29 {
                }
                frame 30 {
                }
                frame 31 {
                  n2278 = property on="FF Calibration g" class="WFGraph (strict)"("X Scale.Name Label.Text"=w3401) -> ()  [unwired: 2 in, 2 out]
                }
                frame 32 {
                  n2279 = property on="RSTCOF" class="Bool"("Boolean Text.Text"=w3402) -> ()  [unwired: 2 in, 2 out]
                  n2280 = property on="RST FF" class="Bool"("Boolean Text.Text"=w3402) -> ()  [unwired: 2 in, 2 out]
                  n2281 = property on="RST TEMP" class="Bool"("Boolean Text.Text"=w3402) -> ()  [unwired: 2 in, 2 out]
                  n2282 = property on="RSTV1 3" class="Bool"("Boolean Text.Text"=w3402) -> ()  [unwired: 2 in, 2 out]
                  n2283 = property on="rstv2" class="Bool"("Boolean Text.Text"=w3402) -> ()  [unwired: 2 in, 2 out]
                  n2284 = property on="RSTV1 2" class="Bool"("Boolean Text.Text"=w3402) -> ()  [unwired: 2 in, 2 out]
                  n2285 = property on="RST CP" class="Bool"("Boolean Text.Text"=w3402) -> ()  [unwired: 2 in, 2 out]
                }
                frame 33 {
                  "S 61" <- w3403
                }
                frame 34 {
                  "String 23" <- w3404
                }
                frame 35 {
                  n2286 = property on="Rh Before" class="DigNum (strict)"("Caption.Text"=w3405) -> ()  [unwired: 2 in, 2 out]
                }
                frame 36 {
                  n2287 = Match Pattern(string=w3406, regular expression=",") -> (before substring=→"bs":string, after substring=→"as":string)  [unwired: 1 in, 2 out]
                  n2288 = property on="Rh After" class="DigNum (strict)"("Caption.Text"=w3406) -> ()  [unwired: 2 in, 2 out]
                }
                frame 37 {
                  n2289 = Match Pattern(string=w3415, regular expression=",") -> (before substring=w3414:string, after substring=w3413:string)  [unwired: 1 in, 2 out]
                  "bs" <- w3414
                  "as" <- w3413
                  n2290 = Concatenate Strings(w3414, w3413) -> (w3410:string)
                  n2291 = property on="Humidity before test 2" class="DigNum (strict)"("Caption.Text"=w3410) -> ()  [unwired: 2 in, 2 out]
                  n2292 = property on="Humidity before test" class="DigNum (strict)"("Caption.Text"=w3410) -> ()  [unwired: 2 in, 2 out]
                  n2293 = Concatenate Strings(w3410, "=" ("string")) -> (w3411:string)
                  n2294 = local write "S 38"(w3411) -> ()
                }
                frame 38 {
                  n2295 = Match Pattern(string=w3422, regular expression=",") -> (before substring=w3421:string, after substring=w3420:string)  [unwired: 1 in, 2 out]
                  "bs" <- w3421
                  "as" <- w3420
                  n2296 = Concatenate Strings(w3421, w3420) -> (w3417:string)
                  n2297 = property on="Humidity after test 2" class="DigNum (strict)"("Caption.Text"=w3417) -> ()  [unwired: 2 in, 2 out]
                  n2298 = Concatenate Strings(w3417, "=" ("string")) -> (w3419:string)
                  n2299 = property on="Humidity after test" class="DigNum (strict)"("Caption.Text"=w3417) -> ()  [unwired: 2 in, 2 out]
                  n2300 = local write "S 39"(w3419) -> ()
                }
                frame 39 {
                  n2301 = Match Pattern(string=w3429, regular expression=",") -> (before substring=w3428:string, after substring=w3427:string)  [unwired: 1 in, 2 out]
                  "bs" <- w3428
                  "as" <- w3427
                  n2302 = Concatenate Strings(w3428, w3427) -> (w3424:string)
                  n2303 = property on="Temperature before test 2" class="DigNum (strict)"("Caption.Text"=w3424) -> ()  [unwired: 2 in, 2 out]
                  n2304 = property on="Temperature before test" class="DigNum (strict)"("Caption.Text"=w3424) -> ()  [unwired: 2 in, 2 out]
                  n2305 = Concatenate Strings(w3424, "=" ("string")) -> (→"String 34":string)
                }
                frame 40 {
                  n2306 = Match Pattern(string=w3436, regular expression=",") -> (before substring=w3435:string, after substring=w3434:string)  [unwired: 1 in, 2 out]
                  "bs" <- w3435
                  "as" <- w3434
                  n2307 = Concatenate Strings(w3435, w3434) -> (w3431:string)
                  n2308 = property on="Temperature after test 2" class="DigNum (strict)"("Caption.Text"=w3431) -> ()  [unwired: 2 in, 2 out]
                  n2309 = Concatenate Strings(w3431, "=" ("string")) -> (→"String 35":string)
                  n2310 = property on="Temperature after test" class="DigNum (strict)"("Caption.Text"=w3431) -> ()  [unwired: 2 in, 2 out]
                }
                frame 41 {
                  n2311 = property on="AVP" class="DigNum (strict)"("Caption.Text"=w3440) -> ()  [unwired: 2 in, 2 out]
                  n2312 = property on="AVP 2" class="DigNum (strict)"("Caption.Text"=w3440) -> ()  [unwired: 2 in, 2 out]
                  n2313 = Concatenate Strings(w3440, "=" ("string")) -> (→"String 36":string)
                }
                frame 42 {
                  n2314 = property on="MWSD" class="DigNum (strict)"("Caption.Text"=w3443) -> ()  [unwired: 2 in, 2 out]
                  n2315 = property on="MWSD 2" class="DigNum (strict)"("Caption.Text"=w3443) -> ()  [unwired: 2 in, 2 out]
                  n2316 = Concatenate Strings(w3443, "=" ("string")) -> (→"String 37":string)
                }
                frame 43 {
                  n2317 = property on="HCF 2" class="DigNum (strict)"("Caption.Text"=w3446) -> ()  [unwired: 2 in, 2 out]
                  n2318 = property on="HCF" class="DigNum (strict)"("Caption.Text"=w3446) -> ()  [unwired: 2 in, 2 out]
                  n2319 = Concatenate Strings(w3446, "=" ("string")) -> (→"String 38":string)
                }
                frame 44 {
                  n2320 = Concatenate Strings(w3448, "=" ("string")) -> (→"String 39":string)
                  n2321 = property on="WS1.4 2" class="DigNum (strict)"("Caption.Text"=w3448) -> ()  [unwired: 2 in, 2 out]
                  n2322 = property on="WS1.4" class="DigNum (strict)"("Caption.Text"=w3448) -> ()  [unwired: 2 in, 2 out]
                }
                frame 45 {
                  n2323 = property on="Save Results" class="Bool (strict)"("Boolean Text.Text"=w3450) -> ()  [unwired: 2 in, 2 out]
                }
                frame 46 {
                  n2324 = local write "S 47"(w3451) -> ()
                }
                frame 47 {
                  n2325 = local write "S 48"(w3452) -> ()
                }
                frame 48 {
                  n2326 = local write "S 49"(w3453) -> ()
                }
                frame 49 {
                  n2327 = local write "S 50"(w3454) -> ()
                }
                frame 50 {
                  n2328 = local write "S 51"(w3455) -> ()
                }
                frame 51 {
                  n2329 = local write "S 52"(w3456) -> ()
                }
                frame 52 {
                  n2330 = local write "S 53"(w3457) -> ()
                }
                frame 53 {
                  n2331 = local write "S 54"(w3458) -> ()
                }
                frame 54 {
                  n2332 = local write "S 55"(w3459) -> ()
                }
                frame 55 {
                  n2333 = local write "S 56"(w3460) -> ()
                }
                frame 56 {
                  n2334 = local write "S 57"(w3461) -> ()
                }
                frame 57 {
                  n2335 = local write "S 58"(w3462) -> ()
                }
                frame 58 {
                  n2336 = local write "S 59"(w3463) -> ()
                }
                frame 59 {
                  n2337 = local write "S 60"(w3464) -> ()
                }
                frame 60 {
                  n2338 = local write "S 62"(w3465) -> ()
                }
                frame 61 {
                  n2339 = local write "S 63"(w3466) -> ()
                }
                frame 62 {
                  n2340 = local write "S 64"(w3467) -> ()
                }
                frame 63 {
                  n2341 = local write "S 65"(w3468) -> ()
                }
                frame 64 {
                  n2342 = local write "S 66"(w3469) -> ()
                }
                frame 65 {
                  n2343 = local write "S 67"(w3470) -> ()
                }
                frame 66 {
                  n2344 = local write "S 68"(w3471) -> ()
                }
                frame 67 {
                  n2345 = local write "S 69"(w3472) -> ()
                }
                frame 68 {
                  n2346 = local write "S 70"(w3473) -> ()
                }
                frame 69 {
                  n2347 = local write "S 71"(w3474) -> ()
                }
                frame 70 {
                  n2348 = local write "S 72"(w3475) -> ()
                }
                frame 71 {
                  n2349 = local write "S 73"(w3476) -> ()
                }
                frame 72 {
                  n2350 = local write "S 74"(w3477) -> ()
                }
                frame 73 {
                  n2351 = local write "S 75"(w3478) -> ()
                }
                frame 74 {
                  n2352 = local write "S 76"(w3479) -> ()
                }
                frame 75 {
                  n2353 = local write "S 77"(w3480) -> ()
                }
                frame 76 {
                  n2354 = local write "S 78"(w3481) -> ()
                }
                frame 77 {
                  n2355 = local write "S 79"(w3482) -> ()
                }
                frame 79 {
                  n2356 = property on="Sample Temperature" class="XYGraph (strict)"("Y Scale.Name Label.Text"=w3483) -> ()  [unwired: 2 in, 2 out]
                }
                frame 80 {
                  n2357 = local write "S 81"(w3484) -> ()
                  n2358 = property on="Humidity" class="XYGraph (strict)"("Y Scale.Name Label.Text"=w3484) -> ()  [unwired: 2 in, 2 out]
                }
                frame 78 {
                  n2359 = property on="Air Temperature" class="XYGraph (strict)"("X Scale.Name Label.Text"=w3485) -> ()  [unwired: 2 in, 2 out]
                  n2360 = property on="Humidity" class="XYGraph (strict)"("X Scale.Name Label.Text"=w3485) -> ()  [unwired: 2 in, 2 out]
                  n2361 = property on="Sample Temperature" class="XYGraph (strict)"("X Scale.Name Label.Text"=w3485) -> ()  [unwired: 2 in, 2 out]
                  n2362 = property on="Coefficient Of Friction" class="XYGraph (strict)"("X Scale.Name Label.Text"=w3485) -> ()  [unwired: 2 in, 2 out]
                }
                frame 81 {
                  n2363 = property on="Air Temperature" class="XYGraph (strict)"("Y Scale.Name Label.Text"=w3486) -> ()  [unwired: 2 in, 2 out]
                }
                frame 82 {
                  n2364 = local write "S 84"(w3487) -> ()
                }
                frame 83 {
                  n2365 = local write "S 85"(w3488) -> ()
                }
                frame 84 {
                  n2366 = local write "S 86"(w3489) -> ()
                }
                frame 85 {
                  n2367 = local write "S 87"(w3490) -> ()
                }
                frame 86 {
                  n2368 = local write "S 88"(w3491) -> ()
                }
                frame 87 {
                  n2369 = property on="FF Calibration g" class="WFGraph (strict)"("Y Scale.Name Label.Text"=w3492) -> ()  [unwired: 2 in, 2 out]
                }
                frame 88 {
                  n2370 = local write "S 90"(w3493) -> ()
                }
                frame 89 {
                  n2371 = local write "S 91"(w3494) -> ()
                }
                frame 90 {
                  n2372 = local write "S 92"(w3495) -> ()
                }
                frame 91 {
                  n2373 = local write "S 93"(w3496) -> ()
                }
                frame 92 {
                  n2374 = local write "S 94"(w3497) -> ()
                }
                frame 93 {
                  n2375 = local write "S 95"(w3498) -> ()
